vi "File - remove err4.vi"(8 "error in (no error)":errorcluster) -> (0 "error out":errorcluster)   [LabVIEW 2014]
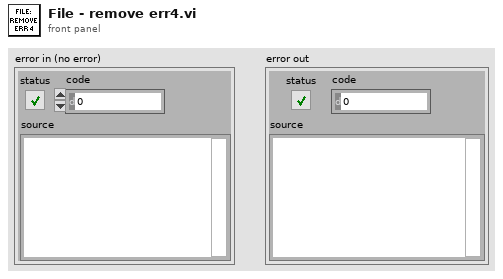
[diagram p1: front panel]
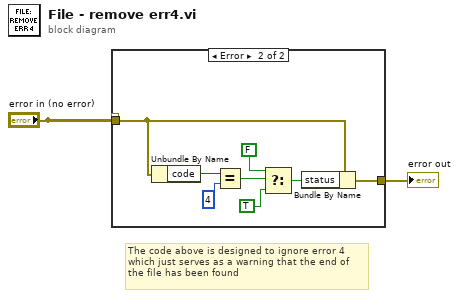
[diagram p0: block diagram]
diagram:
  # "The code above is designed to ignore error 4\nwhich just serves as a warning that the end of\nthe file has been found"
  n1 = case shown="Error" "error in (no error)" {
    selector: "error in (no error)" -> [w3 _]
    tunnel: "error in (no error)" -> [_ w9]
    tunnel: [w3 w4] -> w2
    frame No Error {
    }
    frame Error {
      n2 = Unbundle By Name(w9) -> ("code"=w10:i32)
      n3 = Equal?(x=w10, y=4) -> (x = y?=w6:bool)
      n4 = Select(t=FALSE, s=w6, f=TRUE) -> (s? t:f=w11:bool)
      n5 = Bundle By Name(cluster=w9, "status"=w11) -> (w4:errorcluster)
    }
  }
  "error out" <- w2
